vi "WebView2 Viewer.vi"(2 "ProjectRef":refnum<vi>, 4 "Extra Scripts":string, 5 "FileDependency In":map{path, T1}(c390), 6 "Options":string, 7 "OpenWebBrowser(False)":bool, 8 "error in":errorcluster, 9 "Embedd VISJS Librarya in HTMl File(False)":bool, 10 "HTMLFilePath":path, 11 "LibraryDependency":map{path, T3}(c390)) -> (0 "error out":errorcluster, 3 "HTMLFileContent":string)   [LabVIEW 2020, in "WebView2-Viewer.lvlib"] (continued)
A=this.body.nodes[g].containedNodes;for(var e in A)Object.prototype.hasOwnProperty.call(A,e)&&t.push(this.body.nodes[e].id)}return t}},{key:\"findNode\",value:function(g){for(var t,A=[],e=0;void 0!==this.clusteredNodes[g]&&e<100;){if(void 0===(t=this.body.nodes[g]))return[];A.push(t.id),g=this.clusteredNodes[g].clusterId,e++}return void 0===(t=this.body.nodes[g])?[]:(A.push(t.id),cl(A).call(A),A)}},{key:\"updateClusteredNode\",value:function(g,t){if(void 0===g)throw new Error(\"No clusteredNodeId supplied to updateClusteredNode.\");if(void 0===t)throw new Error(\"No newOptions supplied to updateClusteredNode.\");if(void 0===this.body.nodes[g])throw new Error(\"The clusteredNodeId supplied to updateClusteredNode does not exist.\");this.body.nodes[g].setOptions(t),this.body.emitter.emit(\"_dataChanged\")}},{key:\"updateEdge\",value:function(g,t){if(void 0===g)throw new Error(\"No startEdgeId supplied to updateEdge.\");if(void 0===t)throw new Error(\"No newOptions supplied to updateEdge.\");if(void 0===this.body.edges[g])throw new Error(\"The startEdgeId supplied to updateEdge does not exist.\");for(var A=this.getClusteredEdges(g),e=0;e<A.length;e++){this.body.edges[A[e]].setOptions(t)}this.body.emitter.emit(\"_dataChanged\")}},{key:\"getClusteredEdges\",value:function(g){for(var t=[],A=0;void 0!==g&&void 0!==this.body.edges[g]&&A<100;)t.push(this.body.edges[g].id),g=this.body.edges[g].edgeReplacedById,A++;return cl(t).call(t),t}},{key:\"getBaseEdge\",value:function(g){return this.getBaseEdges(g)[0]}},{key:\"getBaseEdges\",value:function(g){for(var t=[g],A=[],e=[],C=0;t.length>0&&C<100;){var I=t.pop();if(void 0!==I){var i=this.body.edges[I];if(void 0!==i){C++;var o=i.clusteringEdgeReplacingIds;if(void 0===o)e.push(I);else for(var n=0;n<o.length;++n){var r=o[n];-1===Xc(t).call(t,o)&&-1===Xc(A).call(A,o)&&t.push(r)}A.push(I)}}}return e}},{key:\"_getConnectedId\",value:function(g,t){return g.toId!=t?g.toId:(g.fromId,g.fromId)}},{key:\"_getHubSize\",value:function(){for(var g=0,t=0,A=0,e=0,C=0;C<this.body.nodeIndices.length;C++){var I=this.body.nodes[this.body.nodeIndices[C]];I.edges.length>e&&(e=I.edges.length),g+=I.edges.length,t+=Math.pow(I.edges.length,2),A+=1}g/=A;var i=(t/=A)-Math.pow(g,2),o=Math.sqrt(i),n=Math.floor(g+2*o);return n>e&&(n=e),n}},{key:\"_createClusteredEdge\",value:function(g,t,A,e,C){var I=XR.cloneOptions(A,\"edge\");qf(I,e),I.from=g,I.to=t,I.id=\"clusterEdge:\"+rD(),void 0!==C&&qf(I,C);var i=this.body.functions.createEdge(I);return i.clusteringEdgeReplacingIds=[A.id],i.connect(),this.body.edges[i.id]=i,i}},{key:\"_clusterEdges\",value:function(g,t,A,e){if(t instanceof ZR){var C=t,I={};I[C.id]=C,t=I}if(g instanceof jN){var i=g,o={};o[i.id]=i,g=o}if(null==A)throw new Error(\"_clusterEdges: parameter clusterNode required\");for(var n in void 0===e&&(e=A.clusterEdgeProperties),this._createClusterEdges(g,t,A,e),t)if(Object.prototype.hasOwnProperty.call(t,n)&&void 0!==this.body.edges[n]){var r=this.body.edges[n];this._backupEdgeOptions(r),r.setOptions({physics:!1})}for(var s in g)Object.prototype.hasOwnProperty.call(g,s)&&(this.clusteredNodes[s]={clusterId:A.id,node:this.body.nodes[s]},this.body.nodes[s].setOptions({physics:!1}))}},{key:\"_getClusterNodeForNode\",value:function(g){if(void 0!==g){var t=this.clusteredNodes[g];if(void 0!==t){var A=t.clusterId;if(void 0!==A)return this.body.nodes[A]}}}},{key:\"_filter\",value:function(g,t){var A=[];return tv(g,(function(g){t(g)&&A.push(g)})),A}},{key:\"_updateState\",value:function(){var g,t=this,A=[],e={},C=function(g){tv(t.body.nodes,(function(t){!0===t.isCluster&&g(t)}))};for(g in this.clusteredNodes){if(Object.prototype.hasOwnProperty.call(this.clusteredNodes,g))void 0===this.body.nodes[g]&&A.push(g)}C((function(g){for(var t=0;t<A.length;t++)delete g.containedNodes[A[t]]}));for(var I=0;I<A.length;I++)delete this.clusteredNodes[A[I]];tv(this.clusteredEdges,(function(g){var A=t.body.edges[g];void 0!==A&&A.endPointsValid()||(e[g]=g)})),C((function(g){tv(g.containedEdges,(function(g,t){g.endPointsValid()||e[t]||(e[t]=t)}))})),tv(this.body.edges,(function(g,A){var C=!0,I=g.clusteringEdgeReplacingIds;if(void 0!==I){var i=0;tv(I,(function(g){var A=t.body.edges[g];void 0!==A&&A.endPointsValid()&&(i+=1)})),C=i>0}g.endPointsValid()&&C||(e[A]=A)})),C((function(g){tv(e,(function(A){delete g.containedEdges[A],tv(g.edges,(function(C,I){C.id!==A?C.clusteringEdgeReplacingIds=t._filter(C.clusteringEdgeReplacingIds,(function(g){return!e[g]})):g.edges[I]=null})),g.edges=t._filter(g.edges,(function(g){return null!==g}))}))})),tv(e,(function(g){delete t.clusteredEdges[g]})),tv(e,(function(g){delete t.body.edges[g]})),tv(Lh(this.body.edges),(function(g){var A=t.body.edges[g],e=t._isClusteredNode(A.fromId)||t._isClusteredNode(A.toId);if(e!==t._isClusteredEdge(A.id))if(e){var C=t._getClusterNodeForNode(A.fromId);void 0!==C&&t._clusterEdges(t.body.nodes[A.fromId],A,C);var I=t._getClusterNodeForNode(A.toId);void 0!==I&&t._clusterEdges(t.body.nodes[A.toId],A,I)}else delete t._clusterEdges[g],t._restoreEdge(A)}));for(var i=!1,o=!0,n=function(){var g=[];C((function(t){var A=Lh(t.containedNodes).length,e=!0===t.options.allowSingleNodeCluster;(e&&A<1||!e&&A<2)&&g.push(t.id)}));for(var A=0;A<g.length;++A)t.openCluster(g[A],{},!1);o=g.length>0,i=i||o};o;)n();i&&this._updateState()}},{key:\"_isClusteredNode\",value:function(g){return void 0!==this.clusteredNodes[g]}},{key:\"_isClusteredEdge\",value:function(g){return void 0!==this.clusteredEdges[g]}}]),g}();var gP=function(){function g(t,A){var e;cn(this,g),void 0!==window&&(e=window.requestAnimationFrame||window.mozRequestAnimationFrame||window.webkitRequestAnimationFrame||window.msRequestAnimationFrame),window.requestAnimationFrame=void 0===e?function(g){g()}:e,this.body=t,this.canvas=A,this.redrawRequested=!1,this.renderTimer=void 0,this.requiresTimeout=!0,this.renderingActive=!1,this.renderRequests=0,this.allowRedraw=!0,this.dragging=!1,this.zooming=!1,this.options={},this.defaultOptions={hideEdgesOnDrag:!1,hideEdgesOnZoom:!1,hideNodesOnDrag:!1},fe(this.options,this.defaultOptions),this._determineBrowserMethod(),this.bindEventListeners()}return kd(g,[{key:\"bindEventListeners\",value:function(){var g,t=this;this.body.emitter.on(\"dragStart\",(function(){t.dragging=!0})),this.body.emitter.on(\"dragEnd\",(function(){t.dragging=!1})),this.body.emitter.on(\"zoom\",(function(){t.zooming=!0,window.clearTimeout(t.zoomTimeoutId),t.zoomTimeoutId=wu((function(){var g;t.zooming=!1,je(g=t._requestRedraw).call(g,t)()}),250)})),this.body.emitter.on(\"_resizeNodes\",(function(){t._resizeNodes()})),this.body.emitter.on(\"_redraw\",(function(){!1===t.renderingActive&&t._redraw()})),this.body.emitter.on(\"_blockRedraw\",(function(){t.allowRedraw=!1})),this.body.emitter.on(\"_allowRedraw\",(function(){t.allowRedraw=!0,t.redrawRequested=!1})),this.body.emitter.on(\"_requestRedraw\",je(g=this._requestRedraw).call(g,this)),this.body.emitter.on(\"_startRendering\",(function(){t.renderRequests+=1,t.renderingActive=!0,t._startRendering()})),this.body.emitter.on(\"_stopRendering\",(function(){t.renderRequests-=1,t.renderingActive=t.renderRequests>0,t.renderTimer=void 0})),this.body.emitter.on(\"destroy\",(function(){t.renderRequests=0,t.allowRedraw=!1,t.renderingActive=!1,!0===t.requiresTimeout?clearTimeout(t.renderTimer):window.cancelAnimationFrame(t.renderTimer),t.body.emitter.off()}))}},{key:\"setOptions\",value:function(g){if(void 0!==g){Xf([\"hideEdgesOnDrag\",\"hideEdgesOnZoom\",\"hideNodesOnDrag\"],this.options,g)}}},{key:\"_requestNextFrame\",value:function(g,t){if(\"undefined\"!=typeof window){var A,e=window;return!0===this.requiresTimeout?A=wu(g,t):e.requestAnimationFrame&&(A=e.requestAnimationFrame(g)),A}}},{key:\"_startRendering\",value:function(){var g;!0===this.renderingActive&&(void 0===this.renderTimer&&(this.renderTimer=this._requestNextFrame(je(g=this._renderStep).call(g,this),this.simulationInterval)))}},{key:\"_renderStep\",value:function(){!0===this.renderingActive&&(this.renderTimer=void 0,!0===this.requiresTimeout&&this._startRendering(),this._redraw(),!1===this.requiresTimeout&&this._startRendering())}},{key:\"redraw\",value:function(){this.body.emitter.emit(\"setSize\"),this._redraw()}},{key:\"_requestRedraw\",value:function(){var g=this;!0!==this.redrawRequested&&!1===this.renderingActive&&!0===this.allowRedraw&&(this.redrawRequested=!0,this._requestNextFrame((function(){g._redraw(!1)}),0))}},{key:\"_redraw\",value:function(){var g=arguments.length>0&&void 0!==arguments[0]&&arguments[0];if(!0===this.allowRedraw){this.body.emitter.emit(\"initRedraw\"),this.redrawRequested=!1;var t={drawExternalLabels:null};0!==this.canvas.frame.canvas.width&&0!==this.canvas.frame.canvas.height||this.canvas.setSize(),this.canvas.setTransform();var A=this.canvas.getContext(),e=this.canvas.frame.canvas.clientWidth,C=this.canvas.frame.canvas.clientHeight;if(A.clearRect(0,0,e,C),0===this.canvas.frame.clientWidth)return;if(A.save(),A.translate(this.body.view.translation.x,this.body.view.translation.y),A.scale(this.body.view.scale,this.body.view.scale),A.beginPath(),this.body.emitter.emit(\"beforeDrawing\",A),A.closePath(),!1===g&&(!1===this.dragging||!0===this.dragging&&!1===this.options.hideEdgesOnDrag)&&(!1===this.zooming||!0===this.zooming&&!1===this.options.hideEdgesOnZoom)&&this._drawEdges(A),!1===this.dragging||!0===this.dragging&&!1===this.options.hideNodesOnDrag){var I=this._drawNodes(A,g).drawExternalLabels;t.drawExternalLabels=I}!1===g&&(!1===this.dragging||!0===this.dragging&&!1===this.options.hideEdgesOnDrag)&&(!1===this.zooming||!0===this.zooming&&!1===this.options.hideEdgesOnZoom)&&this._drawArrows(A),null!=t.drawExternalLabels&&t.drawExternalLabels(),!1===g&&this._drawSelectionBox(A),A.beginPath(),this.body.emitter.emit(\"afterDrawing\",A),A.closePath(),A.restore(),!0===g&&A.clearRect(0,0,e,C)}}},{key:\"_resizeNodes\",value:function(){this.canvas.setTransform();var g=this.canvas.getContext();g.save(),g.translate(this.body.view.translation.x,this.body.view.translation.y),g.scale(this.body.view.scale,this.body.view.scale);var t,A=this.body.nodes;for(var e in A)Object.prototype.hasOwnProperty.call(A,e)&&((t=A[e]).resize(g),t.updateBoundingBox(g,t.selected));g.restore()}},{key:\"_drawNodes\",value:function(g){for(var t,A,e=arguments.length>1&&void 0!==arguments[1]&&arguments[1],C=this.body.nodes,I=this.body.nodeIndices,i=[],o=[],n=this.canvas.DOMtoCanvas({x:-20,y:-20}),r=this.canvas.DOMtoCanvas({x:this.canvas.frame.canvas.clientWidth+20,y:this.canvas.frame.canvas.clientHeight+20}),s={top:n.y,left:n.x,bottom:r.y,right:r.x},a=[],d=0;d<I.length;d++)if((t=C[I[d]]).hover)o.push(I[d]);else if(t.isSelected())i.push(I[d]);else if(!0===e){var h=t.draw(g);null!=h.drawExternalLabel&&a.push(h.drawExternalLabel)}else if(!0===t.isBoundingBoxOverlappingWith(s)){var l=t.draw(g);null!=l.drawExternalLabel&&a.push(l.drawExternalLabel)}else t.updateBoundingBox(g,t.selected);var c=i.length,u=o.length;for(A=0;A<c;A++){var p=(t=C[i[A]]).draw(g);null!=p.drawExternalLabel&&a.push(p.drawExternalLabel)}for(A=0;A<u;A++){var f=(t=C[o[A]]).draw(g);null!=f.drawExternalLabel&&a.push(f.drawExternalLabel)}return{drawExternalLabels:function(){for(var g=0,t=a;g<t.length;g++){(0,t[g])()}}}}},{key:\"_drawEdges\",value:function(g){for(var t=this.body.edges,A=this.body.edgeIndices,e=0;e<A.length;e++){var C=t[A[e]];!0===C.connected&&C.draw(g)}}},{key:\"_drawArrows\",value:function(g){for(var t=this.body.edges,A=this.body.edgeIndices,e=0;e<A.length;e++){var C=t[A[e]];!0===C.connected&&C.drawArrows(g)}}},{key:\"_determineBrowserMethod\",value:function(){if(\"undefined\"!=typeof window){var g=navigator.userAgent.toLowerCase();this.requiresTimeout=!1,(-1!=Xc(g).call(g,\"msie 9.0\")||-1!=Xc(g).call(g,\"safari\")&&Xc(g).call(g,\"chrome\")<=-1)&&(this.requiresTimeout=!0)}else this.requiresTimeout=!0}},{key:\"_drawSelectionBox\",value:function(g){if(this.body.selectionBox.show){g.beginPath();var t=this.body.selectionBox.position.end.x-this.body.selectionBox.position.start.x,A=this.body.selectionBox.position.end.y-this.body.selectionBox.position.start.y;g.rect(this.body.selectionBox.position.start.x,this.body.selectionBox.position.start.y,t,A),g.fillStyle=\"rgba(151, 194, 252, 0.2)\",g.fillRect(this.body.selectionBox.position.start.x,this.body.selectionBox.position.start.y,t,A),g.strokeStyle=\"rgba(151, 194, 252, 1)\",g.stroke()}else g.closePath()}}]),g}(),tP=A(tg.setInterval);function AP(g,t){t.inputHandler=function(g){g.isFirst&&t(g)},g.on(\"hammer.input\",t.inputHandler)}function eP(g,t){return t.inputHandler=function(g){g.isFinal&&t(g)},g.on(\"hammer.input\",t.inputHandler)}var CP=function(){function g(t){cn(this,g),this.body=t,this.pixelRatio=1,this.cameraState={},this.initialized=!1,this.canvasViewCenter={},this._cleanupCallbacks=[],this.options={},this.defaultOptions={autoResize:!0,height:\"100%\",width:\"100%\"},fe(this.options,this.defaultOptions),this.bindEventListeners()}return kd(g,[{key:\"bindEventListeners\",value:function(){var g,t=this;this.body.emitter.once(\"resize\",(function(g){0!==g.width&&(t.body.view.translation.x=.5*g.width),0!==g.height&&(t.body.view.translation.y=.5*g.height)})),this.body.emitter.on(\"setSize\",je(g=this.setSize).call(g,this)),this.body.emitter.on(\"destroy\",(function(){t.hammerFrame.destroy(),t.hammer.destroy(),t._cleanUp()}))}},{key:\"setOptions\",value:function(g){var t=this;if(void 0!==g){Xf([\"width\",\"height\",\"autoResize\"],this.options,g)}if(this._cleanUp(),!0===this.options.autoResize){var A;if(window.ResizeObserver){var e=new ResizeObserver((function(){!0===t.setSize()&&t.body.emitter.emit(\"_requestRedraw\")})),C=this.frame;e.observe(C),this._cleanupCallbacks.push((function(){e.unobserve(C)}))}else{var I=tP((function(){!0===t.setSize()&&t.body.emitter.emit(\"_requestRedraw\")}),1e3);this._cleanupCallbacks.push((function(){clearInterval(I)}))}var i=je(A=this._onResize).call(A,this);window.addEventListener(\"resize\",i),this._cleanupCallbacks.push((function(){window.removeEventListener(\"resize\",i)}))}}},{key:\"_cleanUp\",value:function(){var g,t,A;Cl(g=cl(t=Zl(A=this._cleanupCallbacks).call(A,0)).call(t)).call(g,(function(g){try{g()}catch(g){console.error(g)}}))}},{key:\"_onResize\",value:function(){this.setSize(),this.body.emitter.emit(\"_redraw\")}},{key:\"_getCameraState\",value:function(){var g=arguments.length>0&&void 0!==arguments[0]?arguments[0]:this.pixelRatio;!0===this.initialized&&(this.cameraState.previousWidth=this.frame.canvas.width/g,this.cameraState.previousHeight=this.frame.canvas.height/g,this.cameraState.scale=this.body.view.scale,this.cameraState.position=this.DOMtoCanvas({x:.5*this.frame.canvas.width/g,y:.5*this.frame.canvas.height/g}))}},{key:\"_setCameraState\",value:function(){if(void 0!==this.cameraState.scale&&0!==this.frame.canvas.clientWidth&&0!==this.frame.canvas.clientHeight&&0!==this.pixelRatio&&this.cameraState.previousWidth>0&&this.cameraState.previousHeight>0){var g=this.frame.canvas.width/this.pixelRatio/this.cameraState.previousWidth,t=this.frame.canvas.height/this.pixelRatio/this.cameraState.previousHeight,A=this.cameraState.scale;1!=g&&1!=t?A=.5*this.cameraState.scale*(g+t):1!=g?A=this.cameraState.scale*g:1!=t&&(A=this.cameraState.scale*t),this.body.view.scale=A;var e=this.DOMtoCanvas({x:.5*this.frame.canvas.clientWidth,y:.5*this.frame.canvas.clientHeight}),C={x:e.x-this.cameraState.position.x,y:e.y-this.cameraState.position.y};this.body.view.translation.x+=C.x*this.body.view.scale,this.body.view.translation.y+=C.y*this.body.view.scale}}},{key:\"_prepareValue\",value:function(g){if(\"number\"==typeof g)return g+\"px\";if(\"string\"==typeof g){if(-1!==Xc(g).call(g,\"%\")||-1!==Xc(g).call(g,\"px\"))return g;if(-1===Xc(g).call(g,\"%\"))return g+\"px\"}throw new Error(\"Could not use the value supplied for width or height:\"+g)}},{key:\"_create\",value:function(){for(;this.body.container.hasChildNodes();)this.body.container.removeChild(this.body.container.firstChild);if(this.frame=document.createElement(\"div\"),this.frame.className=\"vis-network\",this.frame.style.position=\"relative\",this.frame.style.overflow=\"hidden\",this.frame.tabIndex=0,this.frame.canvas=document.createElement(\"canvas\"),this.frame.canvas.style.position=\"relative\",this.frame.appendChild(this.frame.canvas),this.frame.canvas.getContext)this._setPixelRatio(),this.setTransform();else{var g=document.createElement(\"DIV\");g.style.color=\"red\",g.style.fontWeight=\"bold\",g.style.padding=\"10px\",g.innerText=\"Error: your browser does not support HTML canvas\",this.frame.canvas.appendChild(g)}this.body.container.appendChild(this.frame),this.body.view.scale=1,this.body.view.translation={x:.5*this.frame.canvas.clientWidth,y:.5*this.frame.canvas.clientHeight},this._bindHammer()}},{key:\"_bindHammer\",value:function(){var g=this;void 0!==this.hammer&&this.hammer.destroy(),this.drag={},this.pinch={},this.hammer=new Ev(this.frame.canvas),this.hammer.get(\"pinch\").set({enable:!0}),this.hammer.get(\"pan\").set({threshold:5,direction:Ev.DIRECTION_ALL}),AP(this.hammer,(function(t){g.body.eventListeners.onTouch(t)})),this.hammer.on(\"tap\",(function(t){g.body.eventListeners.onTap(t)})),this.hammer.on(\"doubletap\",(function(t){g.body.eventListeners.onDoubleTap(t)})),this.hammer.on(\"press\",(function(t){g.body.eventListeners.onHold(t)})),this.hammer.on(\"panstart\",(function(t){g.body.eventListeners.onDragStart(t)})),this.hammer.on(\"panmove\",(function(t){g.body.eventListeners.onDrag(t)})),this.hammer.on(\"panend\",(function(t){g.body.eventListeners.onDragEnd(t)})),this.hammer.on(\"pinch\",(function(t){g.body.eventListeners.onPinch(t)})),this.frame.canvas.addEventListener(\"wheel\",(function(t){g.body.eventListeners.onMouseWheel(t)})),this.frame.canvas.addEventListener(\"mousemove\",(function(t){g.body.eventListeners.onMouseMove(t)})),this.frame.canvas.addEventListener(\"contextmenu\",(function(t){g.body.eventListeners.onContext(t)})),this.hammerFrame=new Ev(this.frame),eP(this.hammerFrame,(function(t){g.body.eventListeners.onRelease(t)}))}},{key:\"setSize\",value:function(){var g=arguments.length>0&&void 0!==arguments[0]?arguments[0]:this.options.width,t=arguments.length>1&&void 0!==arguments[1]?arguments[1]:this.options.height;g=this._prepareValue(g),t=this._prepareValue(t);var A=!1,e=this.frame.canvas.width,C=this.frame.canvas.height,I=this.pixelRatio;if(this._setPixelRatio(),g!=this.options.width||t!=this.options.height||this.frame.style.width!=g||this.frame.style.height!=t)this._getCameraState(I),this.frame.style.width=g,this.frame.style.height=t,this.frame.canvas.style.width=\"100%\",this.frame.canvas.style.height=\"100%\",this.frame.canvas.width=Math.round(this.frame.canvas.clientWidth*this.pixelRatio),this.frame.canvas.height=Math.round(this.frame.canvas.clientHeight*this.pixelRatio),this.options.width=g,this.options.height=t,this.canvasViewCenter={x:.5*this.frame.clientWidth,y:.5*this.frame.clientHeight},A=!0;else{var i=Math.round(this.frame.canvas.clientWidth*this.pixelRatio),o=Math.round(this.frame.canvas.clientHeight*this.pixelRatio);this.frame.canvas.width===i&&this.frame.canvas.height===o||this._getCameraState(I),this.frame.canvas.width!==i&&(this.frame.canvas.width=i,A=!0),this.frame.canvas.height!==o&&(this.frame.canvas.height=o,A=!0)}return!0===A&&(this.body.emitter.emit(\"resize\",{width:Math.round(this.frame.canvas.width/this.pixelRatio),height:Math.round(this.frame.canvas.height/this.pixelRatio),oldWidth:Math.round(e/this.pixelRatio),oldHeight:Math.round(C/this.pixelRatio)}),this._setCameraState()),this.initialized=!0,A}},{key:\"getContext\",value:function(){return this.frame.canvas.getContext(\"2d\")}},{key:\"_determinePixelRatio\",value:function(){var g=this.getContext();if(void 0===g)throw new Error(\"Could not get canvax context\");var t=1;return\"undefined\"!=typeof window&&(t=window.devicePixelRatio||1),t/(g.webkitBackingStorePixelRatio||g.mozBackingStorePixelRatio||g.msBackingStorePixelRatio||g.oBackingStorePixelRatio||g.backingStorePixelRatio||1)}},
